vi "UploadAndRun.vi"(6 "Python version":string="3.9", 7 "Console":refnum<vi>, 8 "error in":errorcluster, 11 "Arduino in":T1) -> (0 "error out":errorcluster, 1 "Reply":string, 2 "standard error":string, 3 "Arduino out":T1)   [LabVIEW 2022 SP3]
uses:
  ArduinoCtrl.ctl
panel:
  out "resulting string":string
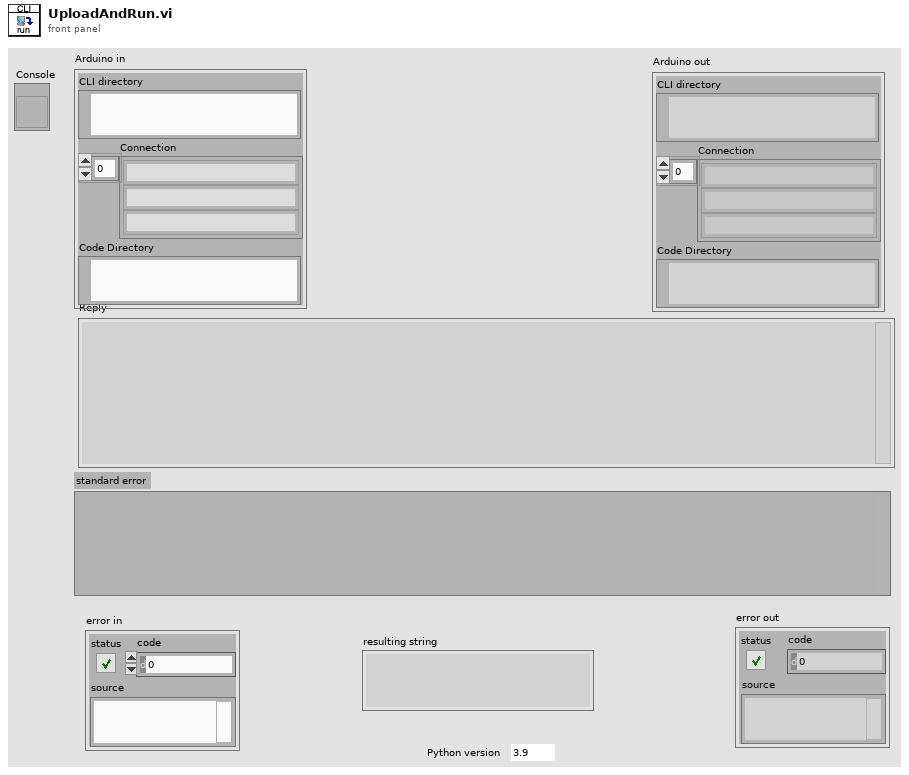
[diagram p1: front panel]
types:
  T1 = typedef "ArduinoCtrl.ctl" = cluster{"CLI directory":path, "Connection":string[], "Code Directory":path}
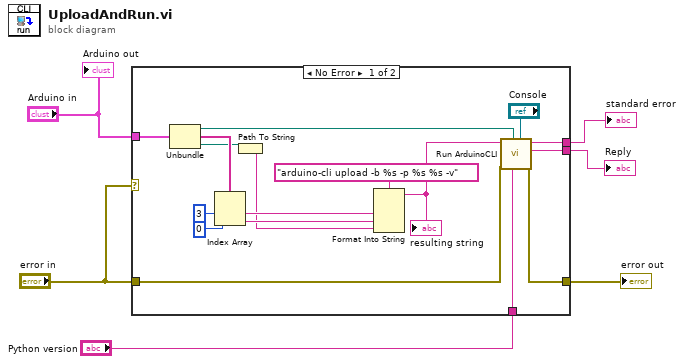
[diagram p0: block diagram]
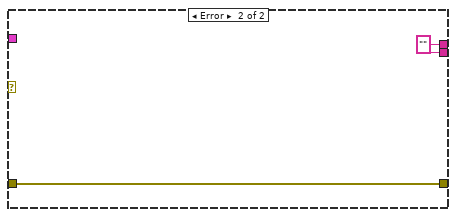
[diagram p2: hidden frame]
diagram:
  n1 = case shown="No Error" "error in" {
    tunnel: "Arduino in" -> [w21 _]
    tunnel: [w20 w25] -> w5
    tunnel: [w19 w25] -> w4
    tunnel: "error in" -> [w11 w24]
    tunnel: [w10 w24] -> w3
    tunnel: "Python version" -> [w7 _]
    frame No Error {
      n2 = Unbundle(w21) -> ("CLI directory"=w12:path, "Connection"=w18:string[], "Code Directory"=w14:path)
      n3 = Index Array(array=w18, index #1=3 ("index"), index #2=0 ("index")) -> (element #1=w16:string, element #2=w15:string)
      n4 = Path To String(path=w14) -> (string=w13:string)
      n5 = Format Into String(format string="arduino-cli upload -b %s -p %s %s -v" ("command line"), w16, w15, w13) -> (resulting string=w22:string)  [unwired: 2 in, 1 out]
      "resulting string" <- w22
      n6 = call "Run ArduinoCLI.vi"("Console"="Console", "Python version"=w7, "working directory"=w12, "error in"=w11, "command line"=w22) -> ("error out"=w10:errorcluster, "standard output"=w19:string, "standard error"=w20:string)  [unwired: 4 in]
    }
    frame Error {
      w25 = "" ("standard error")
    }
  }
  "Reply" <- w4
  "standard error" <- w5
  "error out" <- w3
  "Arduino out" <- "Arduino in"
